vi "EnFlo_CalcTubingCorrection.vi"() -> (5 "Plug in titles":string[](array[string]), 7 "Plug in values":string[](array[string]))   [LabVIEW 2022 SP3]
uses:
  Controls/Setup.ctl
  Globals/Meas_global.vi
panel:
  out "Time dealy in ms":cluster{dbl[], dbl[]}[](graph)
  out "Filename Out":path
  out "Phase Shift":cluster{dbl[], dbl[]}[](graph)
  out "Amplitude Gain":cluster{dbl[], dbl[]}[](graph)
  in  "Test Channel":i32[](listbox)
  in  "Reference Inst":i32(ring) items=["FF1", "FF2", "RV1"]
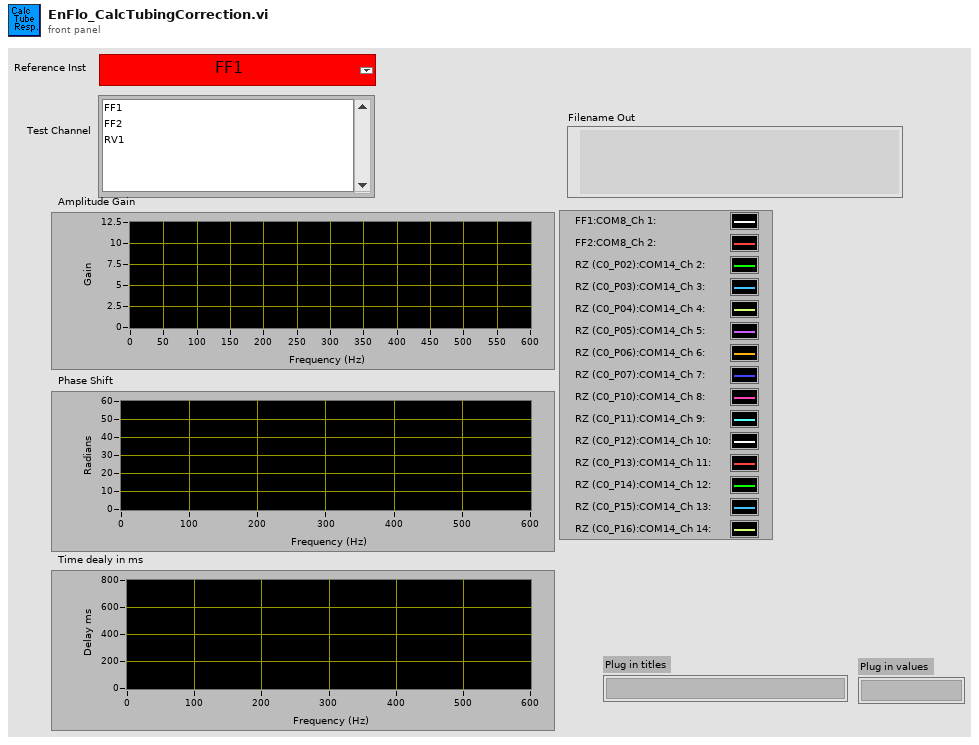
[diagram p1: front panel]
types:
  T1 = typedef "Setup.ctl" = enum16{"Run Program", "Show Setup", "Save Current Setup", "Setup Front Panel"}
  T2 = typedef "Analysis_info_cluster.ctl" = cluster{"Colour":u32, "Inst type":T3, "Inst name":string, "Symbol":string, "Code name":string, "Extra Info":string, "Inst Array":T4, "Extra Titles":string[], "Extra Values":string[], "U":dbl, "u^2":dbl, "u^3":dbl, "u^4":dbl, "Skew_u":dbl, "Kurt_u":dbl, "Sd Error in Mean":dbl, "% u'/U":dbl, "X":dbl, "Y":dbl, "Z":dbl, "Timescale integral Estimate":dbl, "Sd Error in Variance":dbl, "Calib File":path, "Calib Constants":dbl[], "Output Position":bool, "Stats":enum16{"None", "Basic", "Full"}, "Av Sampling Rate":dbl, "Av No of Samples":dbl, "Total Meas Time (s)":dbl, "ADAM Ch Name":string, "Max value":dbl, "Min value":dbl, "Req Sample Rate Hz":dbl, "Sync Delay Time (s)":dbl, "Ch No":i16, "Device":string, "Use Latest Calib":bool, "Port":string, "Metadata Ch Names":string[], "Metadata Ch Values":string[], "Label":string}
  T3 = typedef "Inst_type.ctl" = enum16{"Raw voltage", "Raw with zero offsetting", "Propeller anemometer", "Pressure Transducer", "Pitot-static tube", "Hot wire", "Cross wire 1", "Cross wire 2", "Generic Linear", "Generic Polynomial", "Generic BackPoly", "Fast FID", "Thermocouple", "Cold wire", "Pulsed Wire", "LDA Vel", "LDA Tran time", "LDA Arr time", "Microphone"}
  T4 = typedef "Instrument_Array.ctl" = enum16{"PWA", "LDA", "Analogue"}
  T5 = enum16{"Save no data", "Save data in new files", "Save data in existing files"}
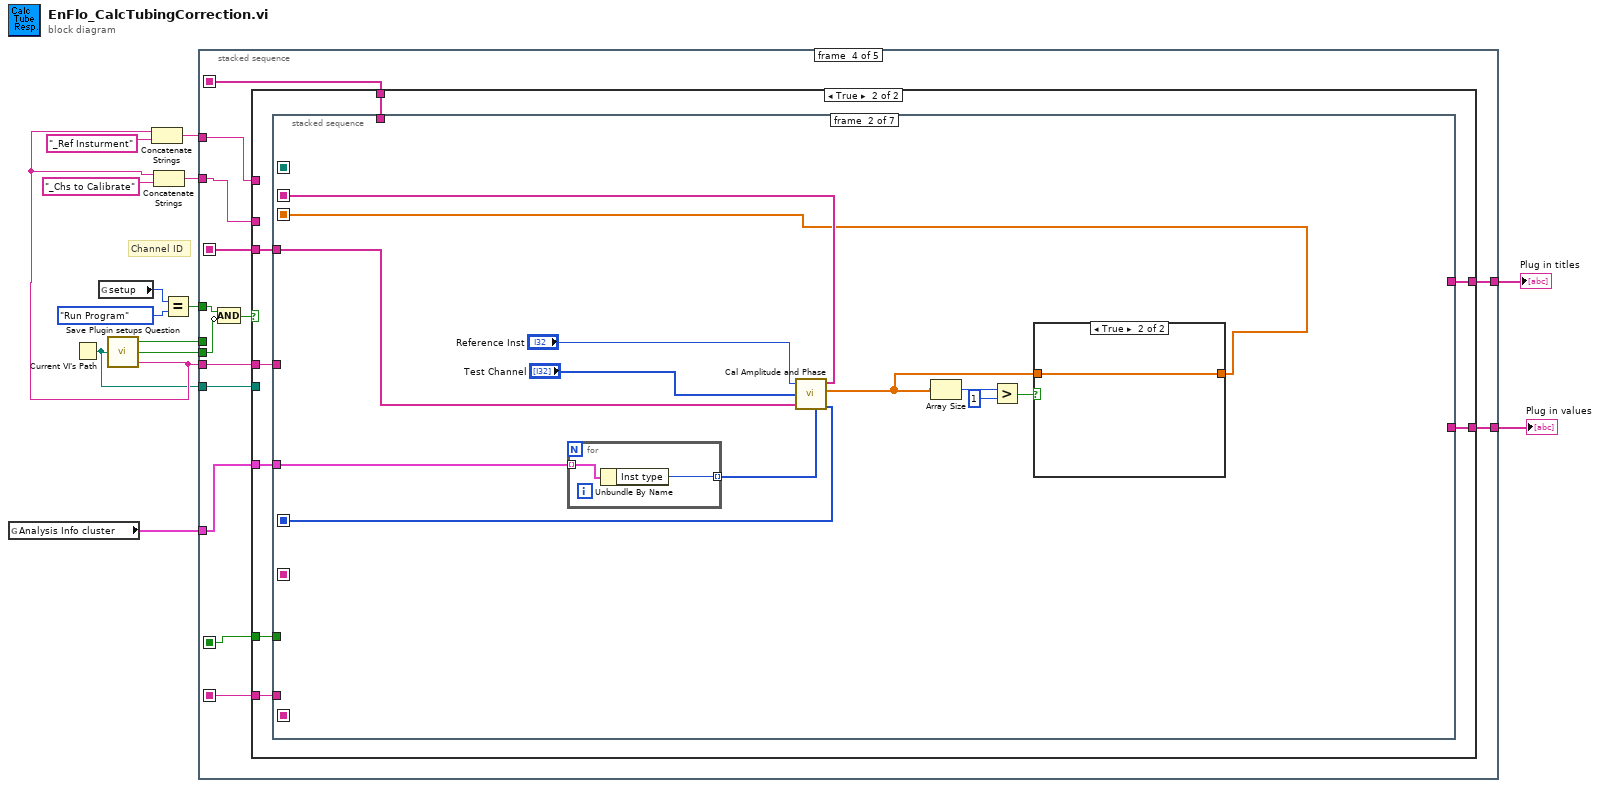
[diagram p0: block diagram]
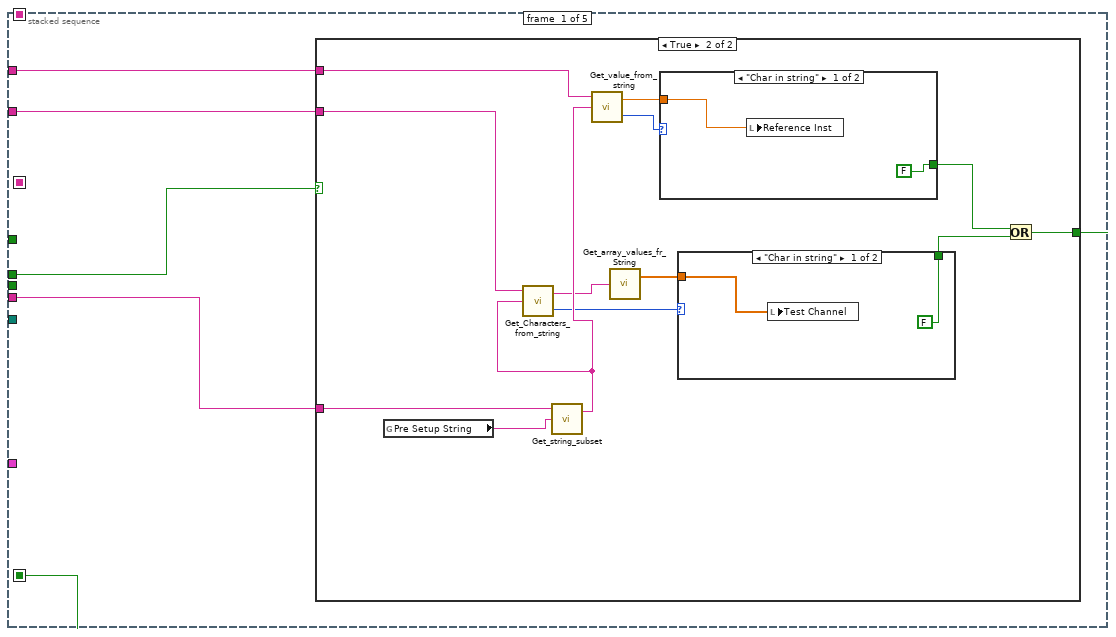
[diagram p2: hidden frame]
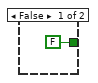
[diagram p3: hidden frame]
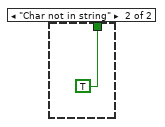
[diagram p4: hidden frame]
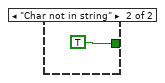
[diagram p5: hidden frame]
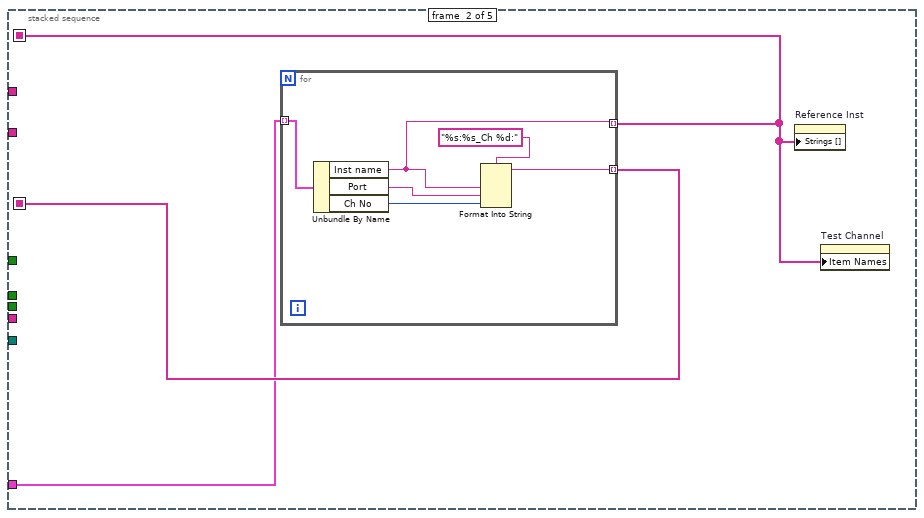
[diagram p6: hidden frame]
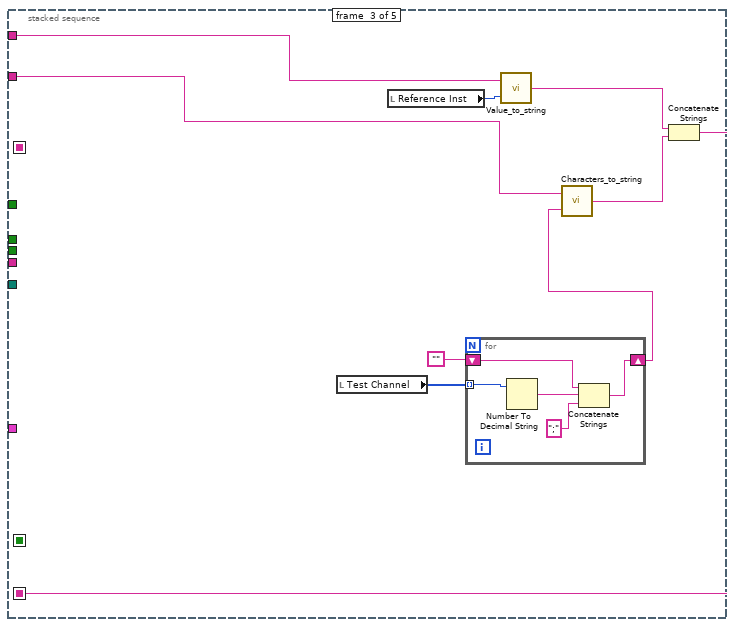
[diagram p7: hidden frame]
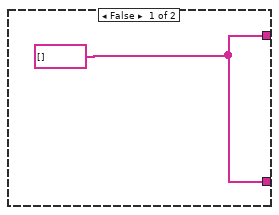
[diagram p8: hidden frame]
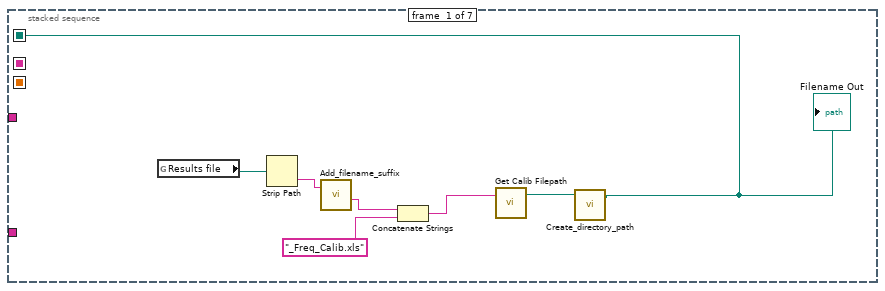
[diagram p9: hidden frame]
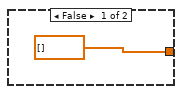
[diagram p10: hidden frame]
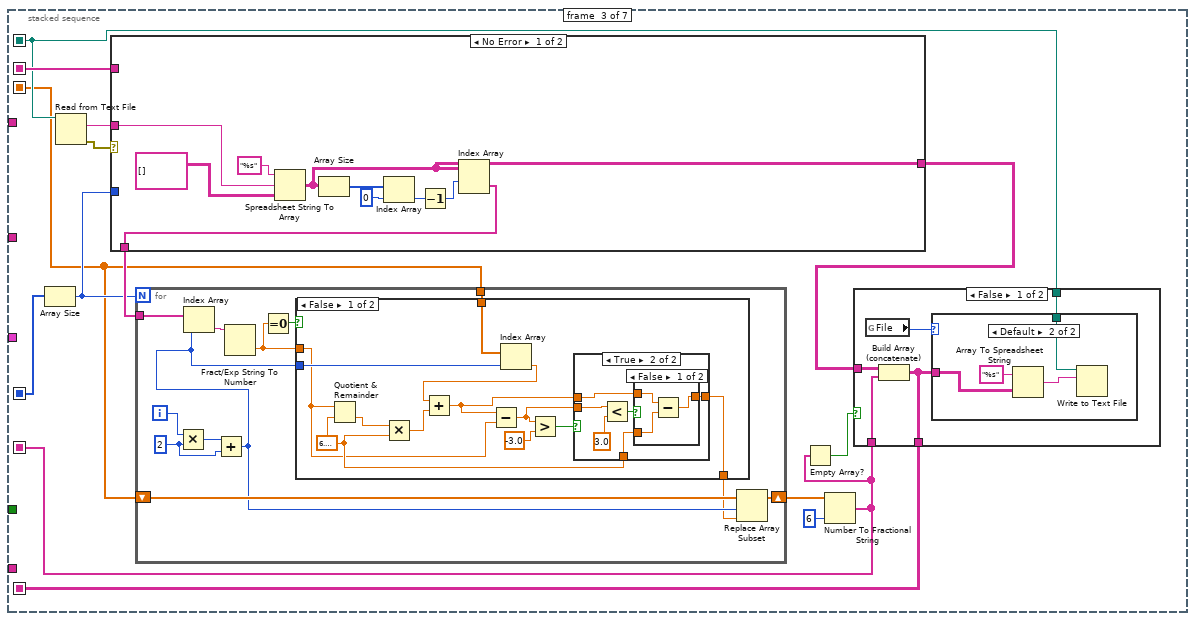
[diagram p11: hidden frame]
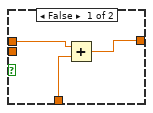
[diagram p14: hidden frame]
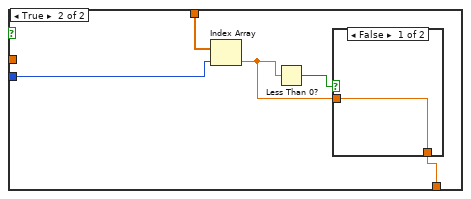
[diagram p16: hidden frame]
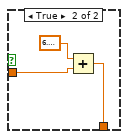
[diagram p17: hidden frame]
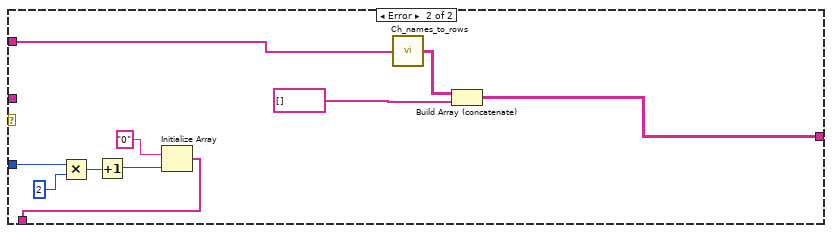
[diagram p18: hidden frame]
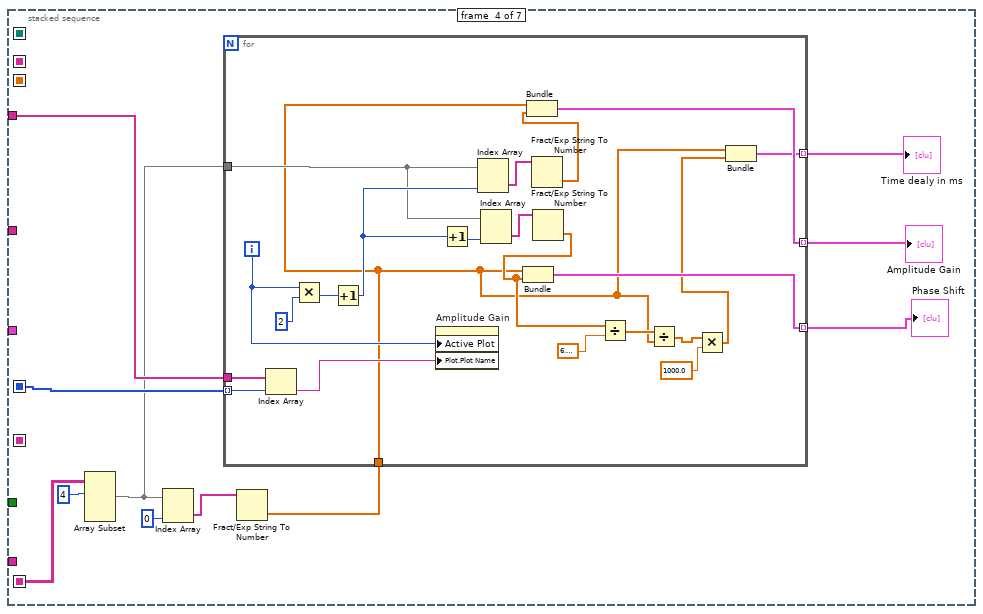
[diagram p19: hidden frame]
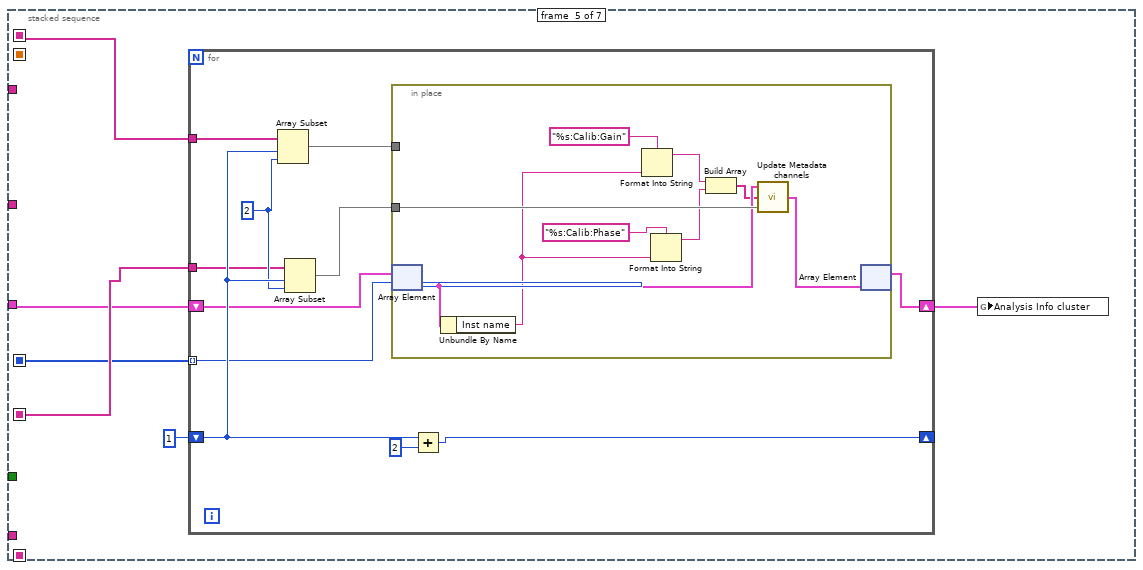
[diagram p20: hidden frame]
diagram:
  # "Channel ID"
  n1 = global read "Meas_global.vi" "Analysis Info cluster"() -> (w3:T2[])
  n2 = Current VI's Path() -> (path=w7:path)
  n3 = global read "Meas_global.vi" "setup"() -> (w5:T1)
  n4 = call "Save Plugin setups Question.vi"("VI path"=w7) -> ("Load Plugin Setup"=w14:bool, "Save Plugin Setup"=w8:bool, "Plugin_Label"=w10:string)
  n5 = Concatenate Strings(w10, "_Ref Insturment" ("string")) -> (w12:string)
  n6 = Concatenate Strings(w10, "_Chs to Calibrate" ("string")) -> (w9:string)
  n7 = Equal?(x=w5, y=Setup."Run Program" ("setup")) -> (x = y?=w4:bool)
  n8 = stacked-sequence {
    seq-local: [_ w42 _ _ _] -> [_ _ _ w73 w274]
    seq-local: [_ w41 _ _ _] -> [_ _ _ w71 w272]
    seq-local: [w15 _ _ _ _] -> [_ _ _ w69 w270]
    seq-local: [_ _ w49 _ _] -> [_ _ _ w70 w271]
    tunnel: w14 -> [w19 _ _ _ _]
    tunnel: w10 -> [w18 _ _ w74 w275]
    tunnel: w12 -> [w17 _ w51 w75 w276]
    tunnel: w9 -> [w16 _ w50 w76 w277]
    tunnel: w8 -> [_ _ _ w68 w278]
    tunnel: w7 -> [_ _ _ w72 w273]
    tunnel: w4 -> [_ _ _ w67 _]
    tunnel: w3 -> [_ w40 _ w65 _]
    tunnel: [_ _ _ w64 _] -> w2
    tunnel: [_ _ _ w63 _] -> w1
    frame #0 {
      n9 = case shown="True" w19 {
        tunnel: w18 -> [_ w32]
        tunnel: w17 -> [_ w31]
        tunnel: w16 -> [_ w28]
        tunnel: [FALSE w21] -> w15
        frame False {
        }
        frame True {
          n10 = global read "Meas_global.vi" "Pre Setup String"() -> (w33:string)
          n11 = call "Get_string_subset.vi"("String to split"=w33, "File Label"=w32) -> ("Output string"=w27:string)  [unwired: 2 in, 1 out]
          n12 = call "Get_Characters_from_string.vi"("Input string"=w27, "Variable name"=w28) -> ("Status"=w25:enum16{"Char in string", "Char not in string"}, "Value"=w26:string)  [unwired: 1 in]
          n13 = call "Get_value_from_string.vi"("Input string"=w27, "Variable name"=w31) -> ("Status"=w30:enum16{"Char in string", "Char not in string"}, "Value"=w29:dbl)  [unwired: 1 in]
          n14 = call "Get_array_values_fr_String.vi"("String Value"=w26) -> ("Numeric Array"=w24:dbl[])  [unwired: 1 out]
          n15 = case shown="\"Char in string\"" w30 {
            tunnel: w29 -> [w38 _]
            tunnel: [FALSE TRUE] -> w23
            frame "Char in string" {
              n16 = local write "Reference Inst"(w38) -> ()
            }
            frame "Char not in string" {
            }
          }
          n17 = case shown="\"Char in string\"" w25 {
            tunnel: w24 -> [w35 _]
            tunnel: [FALSE TRUE] -> w22
            frame "Char in string" {
              n18 = local write "Test Channel"(w35) -> ()
            }
            frame "Char not in string" {
            }
          }
          n19 = Or(x=w23, y=w22) -> (x .or. y?=w21:bool)
        }
      }
    }
    frame #1 {
      n20 = for {
        tunnel: w40 -> [w45] mode=indexing
        tunnel: [w44] -> w42 mode=indexing
        tunnel: [w43] -> w41 mode=indexing
        n21 = Unbundle By Name(w45) -> ("Inst name"=w44:string, "Port"=w46:string, "Ch No"=w47:i16)
        n22 = Format Into String(format string="%s:%s_Ch %d:", w44, w46, w47) -> (resulting string=w43:string)  [unwired: 2 in, 1 out]
      }
      n23 = property on="Reference Inst" class="Ring (strict)"("Strings []"=w42) -> ()  [unwired: 2 in, 2 out]
      n24 = property on="Test Channel" class="LstBox (strict)"("Item Names"=w42) -> ()  [unwired: 2 in, 2 out]
    }
    frame #2 {
      n25 = local read "Test Channel"() -> (w55:i32[])
      n26 = local read "Reference Inst"() -> (w57:i32)
      n27 = for {
        tunnel: w55 -> [w62] mode=indexing
        shift-right: [w58] -> w54
        shift-left: "" -> [w59]
        n28 = Number To Decimal String(number=w62) -> (decimal integer string=w61:string)  [unwired: 1 in]
        n29 = Concatenate Strings(w59, w61, ";" ("string")) -> (w58:string)
      }
      n30 = call "Value_to_string.vi"("Value"=w57, "Label for value"=w51) -> ("Output string"=w56:string)  [unwired: 1 in]
      n31 = call "Characters_to_string.vi"("Characters to write"=w54, "Label for characters"=w50) -> ("Output string"=w53:string)  [unwired: 1 in]
      n32 = Concatenate Strings(w56, w53) -> (w49:string)
    }
    frame #3 {
      n33 = Compound Arithmetic op=AND(w67, invert w68) -> (w66:bool)
      n34 = case shown="True" w66 {
        tunnel: w76 -> [_ _]
        tunnel: w75 -> [_ _]
        tunnel: w74 -> [_ w81]
        tunnel: w73 -> [_ w85]
        tunnel: w72 -> [_ _]
        tunnel: w71 -> [_ w84]
        tunnel: w70 -> [_ w83]
        tunnel: w69 -> [_ w82]
        tunnel: w65 -> [_ w80]
        tunnel: [w77 w79] -> w64
        tunnel: [w77 w78] -> w63
        frame False {
          w77 = string[] [] ("Plug in titles")
        }
        frame True {
          n35 = stacked-sequence {
            seq-local: [w86 _ _ _ _ _ _] -> [_ _ w121 _ _ _ _]
            seq-local: [_ w103 _ _ _ _ _] -> [_ _ w122 _ w235 w262 _]
            seq-local: [_ w94 _ _ _ _ _] -> [_ _ w112 _ _ _ _]
            seq-local: [_ _ w116 _ _ _ _] -> [_ _ _ w206 _ _ _]
            seq-local: [_ w101 _ _ _ _ _] -> [_ _ w114 w204 w232 _ _]
            seq-local: [_ _ w110 _ _ _ _] -> [_ _ _ _ w234 w261 _]
            tunnel: w85 -> [_ _ _ _ _ _ _]
            tunnel: w84 -> [_ w104 _ w203 _ _ _]
            tunnel: w83 -> [_ _ _ _ _ _ w265]
            tunnel: w82 -> [_ _ _ _ _ _ w264]
            tunnel: w81 -> [_ _ _ _ _ _ w263]
            tunnel: w80 -> [_ w99 _ _ w233 _ _]
            tunnel: [_ _ _ _ _ w258 _] -> w79
            tunnel: [_ _ _ _ _ w257 _] -> w78
            frame #0 {
              n36 = global read "Meas_global.vi" "Results file"() -> (w91:path)
              n37 = Strip Path(path=w91) -> (name=w90:string)  [unwired: 1 out]
              n38 = call "Add_filename_suffix.vi"("Filename"=w90) -> ("Base name"=w89:string)  [unwired: 1 in, 3 out]
              n39 = Concatenate Strings(w89, "_Freq_Calib.xls" ("string")) -> (w88:string)
              n40 = call "Get Calib Filepath.vi"("Filename String"=w88) -> ("Filename Out"=w87:path)  [unwired: 2 in]
              n41 = call "Create_directory_path.vi"("Path name"=w87) -> ("Path name Out"=w86:path)  [unwired: 2 in, 1 out]
              "Filename Out" <- w86
            }
            frame #1 {
              n42 = for {
                tunnel: [w108] -> w98 mode=indexing
                tunnel: w99 -> [w107] mode=indexing
                n43 = Unbundle By Name(w107) -> ("Inst type"=w108:T3)
              }
              n44 = call "Cal Amplitude and Phase.vi"("Inst Types"=w98, "Channel ID"=w104, "Test Ch Indices"="Test Channel", "Reference Ch Index"="Reference Inst") -> ("Valid Indices"=w101:i32[], "Ch Values"=w93:dbl[], "Ch Names"=w103:string[])  [unwired: 2 in]
              n45 = Array Size(array=w93) -> (size(s)=w97:i32)
              n46 = Greater?(x=w97, y=1) -> (0:w95:bool)
              n47 = case shown="True" w95 {
                tunnel: [dbl[] [] ("Ch Values") w106] -> w94
                tunnel: w93 -> [_ w106]
                frame False {
                }
                frame True {
                }
              }
            }
            frame #2 {
              n48 = Array Size(array=w114) -> (size(s)=w113:i32)
              n49 = Read from Text File(file (use dialog)=w121) -> (text=w120:string, error out=w119:errorcluster)  [unwired: 3 in, 2 out]
              n50 = case shown="No Error" w119 {
                tunnel: [w180 w194] -> w117
                tunnel: w122 -> [_ w195]
                tunnel: w120 -> [w181 _]
                tunnel: [w179 w188] -> w115
                tunnel: w113 -> [_ w193]
                frame No Error {
                  n51 = Spreadsheet String To Array(format string="%s", spreadsheet string=w181, array type (2D Dbl)=string[][] []) -> (array=w180:string[][])  [unwired: 1 in]
                  n52 = Array Size(array=w180) -> (size(s)=w182:i32[])
                  n53 = Index Array(array=w182, index=0) -> (element=w184:i32)
                  n54 = Decrement(x=w184) -> (x-1=w183:i32)
                  n55 = Index Array(array=w180, index (row)=w183) -> (element=w179:string[])  [unwired: 1 in]
                }
                frame Error {
                  n56 = Multiply(x=w193, y=2) -> (x*y=w191:i32)
                  n57 = Increment(x=w191) -> (x+1=w190:i32)
                  n58 = Initialize Array("0", w190) -> (w188:string[])
                  n59 = call "Ch_names_to_rows.vi"("Channel Names"=w195) -> ("3 Row names"=w196:string[][])
                  n60 = Build Array (concatenate)(w196, string[] [] ("element")) -> (w194:string[][])
                }
              }
              n61 = for {
                N: w113 -> [_]
                tunnel: w112 -> [w140]
                tunnel: w115 -> [w139]
                shift-right: [w136] -> w111
                shift-left: w112 -> [w138]
                i -> [w144]
                w142 = 2 ("y")
                n62 = Multiply(x=w144, y=w142) -> (x*y=w143:i32)
                n63 = Add(x=w143, y=w142) -> (x+y=w137:i32)
                n64 = Index Array(array=w139, index=w137) -> (element=w141:string)
                n65 = Fract/Exp String To Number(string=w141) -> (number=w134:dbl)  [unwired: 3 in, 1 out]
                n66 = Equal To 0?(x=w134) -> (x = 0?=w133:bool)
                n67 = case shown="False" w133 {
                  tunnel: w140 -> [w149 w174]
                  tunnel: w137 -> [w147 w173]
                  tunnel: [w146 w170] -> w135
                  tunnel: w134 -> [w145 _]
                  frame False {
                    w151 = 6.283185307179586
                    n68 = Quotient & Remainder(x=w145, y=w151) -> (floor(x/y)=w152:dbl)  [unwired: 1 out]
                    n69 = Multiply(x=w152, y=w151) -> (x*y=w153:dbl)
                    n70 = Index Array(array=w149, index=w147) -> (element=w148:dbl)
                    n71 = Add(x=w148, y=w153) -> (x+y=w155:dbl)
                    n72 = Subtract(x=w155, y=w145) -> (x-y=w156:dbl)
                    n73 = Greater?(x=w156, y=-3.0) -> (0:w154:bool)
                    n74 = case shown="True" w154 {
                      tunnel: [w157 w161] -> w146
                      tunnel: w155 -> [w158 w162]
                      tunnel: w151 -> [w159 w163]
                      tunnel: w156 -> [_ w160]
                      frame False {
                        n75 = Add(x=w158, y=w159) -> (x+y=w157:dbl)
                      }
                      frame True {
                        n76 = Less?(x=w160, y=3.0) -> (x < y?=w164:bool)
                        n77 = case shown="False" w164 {
                          tunnel: w163 -> [w168 _]
                          tunnel: w162 -> [w167 w169]
                          tunnel: [w166 w169] -> w161
                          frame False {
                            n78 = Subtract(x=w167, y=w168) -> (x-y=w166:dbl)
                          }
                          frame True {
                          }
                        }
                      }
                    }
                  }
                  frame True {
                    n79 = Index Array(array=w174, index=w173) -> (element=w171:dbl)
                    n80 = Less Than 0?(x=w171) -> (x < 0?=w172:bool)
                    n81 = case shown="False" w172 {
                      tunnel: w171 -> [w175 w177]
                      tunnel: [w175 w176] -> w170
                      frame False {
                      }
                      frame True {
                        n82 = Add(x=6.283185307179586, y=w177) -> (x+y=w176:dbl)
                      }
                    }
                  }
                }
                n83 = Replace Array Subset(array=w138, new element=w135, index=w137) -> (w136:dbl[])
              }
              n84 = Number To Fractional String(number=w111, precision (6)=i16 6) -> (F-format string=w110:string[])  [unwired: 2 in]
              n85 = Empty Array?(array=w110) -> (empty?=w109:bool)
              n86 = case shown="False" w109 {
                tunnel: w121 -> [w127 _]
                tunnel: w117 -> [w126 w132]
                tunnel: [w125 w132] -> w116
                tunnel: w110 -> [w123 _]
                frame False {
                  n87 = global read "Meas_global.vi" "File"() -> (w124:T5)
                  n88 = Build Array (concatenate)(w126, w123) -> (w125:string[][])
                  n89 = case shown="Default" w124 {
                    tunnel: w127 -> [_ w129]
                    tunnel: w125 -> [_ w128]
                    frame "Save no data" {
                    }
                    frame Default {
                      n90 = Array To Spreadsheet String(array=w128, 3:"%s" ("format string")) -> (spreadsheet string=w130:string)  [unwired: 1 in]
                      n91 = Write to Text File(file (use dialog)=w129, text=w130) -> ()  [unwired: 2 in, 3 out]
                    }
                  }
                }
                frame True {
                }
              }
            }
            frame #3 {
              n92 = Array Subset(array=w206, index (row)=4 ("index")) -> (w199:string[][])  [unwired: 3 in]
              n93 = Index Array(array=w199, index (col)=0 ("disabled index (col)")) -> (element=w201:string[])  [unwired: 1 in]
              n94 = Fract/Exp String To Number(string=w201) -> (number=w200:dbl[])  [unwired: 3 in, 1 out]
              n95 = for {
                tunnel: [w219] -> w208 mode=indexing
                tunnel: [w220] -> w207 mode=indexing
                tunnel: w204 -> [w230] mode=indexing
                tunnel: w203 -> [w229]
                tunnel: w200 -> [w213]
                tunnel: w199 -> [w224]
                tunnel: [w212] -> w198 mode=indexing
                i -> [w217]
                n96 = Index Array(array=w229, index=w230) -> (element=w228:string)
                n97 = Multiply(x=w217, y=2) -> (x*y=w226:i32)
                n98 = Increment(x=w226) -> (x+1=w225:i32)
                n99 = property on="Amplitude Gain" class="XYGraph (strict)"("Active Plot"=w217, "Plot.Plot Name"=w228) -> ()  [unwired: 2 in, 2 out]
                n100 = Increment(x=w225) -> (x+1=w218:i32)
                n101 = Index Array(array=w224, index (col)=w225) -> (element=w222:string[])  [unwired: 1 in]
                n102 = Index Array(array=w224, index (col)=w218) -> (element=w223:string[])  [unwired: 1 in]
                n103 = Fract/Exp String To Number(string=w222) -> (number=w221:dbl[])  [unwired: 3 in, 1 out]
                n104 = Bundle(w213, w221) -> (w219:cluster{dbl[], dbl[]})  [unwired: 1 in]
                n105 = Fract/Exp String To Number(string=w223) -> (number=w216:dbl[])  [unwired: 3 in, 1 out]
                n106 = Bundle(w213, w216) -> (w220:cluster{dbl[], dbl[]})  [unwired: 1 in]
                n107 = Divide(x=w216, y=6.283185307179586) -> (x/y=w214:dbl[])
                n108 = Divide(x=w214, y=w213) -> (x/y=w211:dbl[])
                n109 = Multiply(x=w211, y=1000.0) -> (x*y=w209:dbl[])
                n110 = Bundle(w213, w209) -> (w212:cluster{dbl[], dbl[]})  [unwired: 1 in]
              }
              "Amplitude Gain" <- w208
              "Phase Shift" <- w207
              "Time dealy in ms" <- w198
            }
            frame #4 {
              n111 = for {
                shift-right: [w246] -> _
                shift-left: 1 -> [w244]
                tunnel: w235 -> [w245]
                tunnel: w234 -> [w242]
                shift-right: [w238] -> w231
                shift-left: w233 -> [w240]
                tunnel: w232 -> [w239] mode=indexing
                w243 = 2 ("length")
                n112 = Array Subset(array=w245, index=w244, length=w243) -> (w237:string[])
                n113 = Array Subset(array=w242, index=w244, length=w243) -> (w241:string[])
                n114 = in-place {
                  in-place-border: w241 -> [w256]
                  in-place-border: w237 -> [_]
                  n115 = in-place-array #1(w240, w239) -> (w254:T2)
                  n116 = Unbundle By Name(w254) -> ("Inst name"=w251:string)
                  n117 = Format Into String(format string="%s:Calib:Gain", w251) -> (resulting string=w250:string)  [unwired: 2 in, 1 out]
                  n118 = Format Into String(format string="%s:Calib:Phase", w251) -> (resulting string=w249:string)  [unwired: 2 in, 1 out]
                  n119 = Build Array(w250, w249) -> (w248:string[])
                  n120 = call "Update Metadata channels.vi"("Metadata Values"=w256, "Metadata Names"=w248, "Analysis info Cluster in"=w254) -> ("Analysis info Cluster out"=w255:T2)
                  n121 = in-place-array #1(w255) -> (w238:T2[])  [unwired: 1 out]
                }
                n122 = Add(x=w244, y=2) -> (x+y=w246:i32)
              }
              n123 = global write "Meas_global.vi" "Analysis Info cluster"(w231) -> ()
            }
            frame #5 {
              n124 = Index Array(array=w262) -> (element=w260:string)  [unwired: 1 in]
              n125 = Index Array(array=w261) -> (element=w259:string)  [unwired: 1 in]
              n126 = Build Array(w260) -> (w257:string[])
              n127 = Build Array(w259) -> (w258:string[])
            }
            frame #6 {
              n128 = case shown="True" w264 {
                tunnel: w265 -> [_ w269]
                tunnel: w263 -> [_ w268]
                frame False {
                }
                frame True {
                  n129 = global read "Meas_global.vi" "New Setup String"() -> (w266:string)
                  n130 = call "Replace_data_in_Label_str.vi"("New data string"=w269, "Input string"=w266, "Variable name"=w268) -> ("Appended string"=w267:string)
                  n131 = global write "Meas_global.vi" "New Setup String"(w267) -> ()
                }
              }
            }
          }
        }
      }
    }
    frame #4 {
      n132 = case shown="True" w278 {
        tunnel: w277 -> [_ _]
        tunnel: w276 -> [_ _]
        tunnel: w275 -> [_ w281]
        tunnel: w274 -> [_ _]
        tunnel: w273 -> [_ w280]
        tunnel: w272 -> [_ _]
        tunnel: w271 -> [_ w279]
        tunnel: w270 -> [_ _]
        frame False {
        }
        frame True {
          n133 = call "Save Plugin Setup String.vi"("Plug In Pathname"=w280, "Setup String to Save"=w279, "PlugIn Label"=w281) -> ()  [unwired: 1 in, 1 out]
        }
      }
    }
  }
  "Plug in titles" <- w1
  "Plug in values" <- w2
